vi "addNode.vi"(0 "reference":refnum<class "ImplicitParameterNode.lvclass">, 1 "node":refnum<class "AbstractNode.lvclass">, 2 "point2D":T1 {"y" format="%.2f"; "x" format="%.2f"}, 5 "error in (no error)":errorcluster) -> (14 "reference out":refnum<class "ImplicitParameterNode.lvclass">, 15 "add":bool, 19 "error out":errorcluster)   [LabVIEW 2014, in "ImplicitParameterNode.lvclass"]
doc: "public boolean addNode(Node n, Point2D p)"
uses:
  <resource>/Framework/Providers/Open_GDS/UML/ImplicitParameterNode_class/ImplicitParameterNode.lvclass
  <resource>/Framework/Providers/Open_GDS/UML/AbstractNode_class/AbstractNode.lvclass
  <resource>/Framework/Providers/Open_GDS/UML/General/Point/Point Point2D.ctl
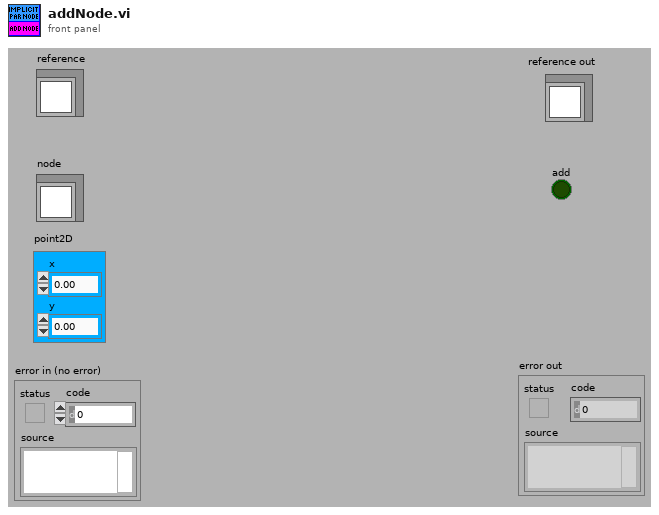
[diagram p1: front panel]
types:
  T1 = typedef "Point Point2D.ctl" = cluster{"x":dbl, "y":dbl}
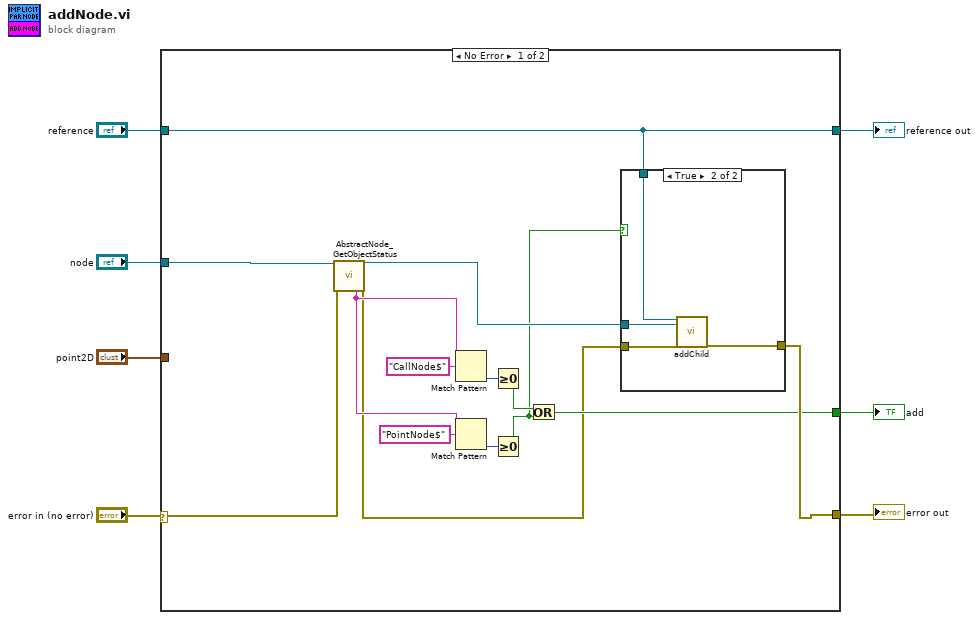
[diagram p0: block diagram]
diagram:
  n1 = case shown="No Error" "error in (no error)" {
    selector: "error in (no error)" -> [w19 w27]
    tunnel: "reference" -> [w21 w28]
    tunnel: [w20 w27] -> w6
    tunnel: [w21 w28] -> w5
    tunnel: "node" -> [w18 _]
    tunnel: "point2D" -> [_ _]
    tunnel: [w17 _] -> w1
    frame No Error {
      n2 = call <resource>:"AbstractNode_GetObjectStatus.vi"("reference in"=w18, "error in (no error)"=w19) -> ("Class name"=w14:string, "reference out"=w9:refnum<class "AbstractNode.lvclass">, "error out"=w10:errorcluster)  [unwired: 15 out]
      n3 = Match Pattern(string=w14, regular expression="CallNode$") -> (offset past match=w13:i32)  [unwired: 4 out]
      n4 = Match Pattern(string=w14, regular expression="PointNode$") -> (offset past match=w12:i32)  [unwired: 4 out]
      n5 = Greater Or Equal To 0?(x=w13) -> (x >= 0?=w11:bool)
      n6 = Greater Or Equal To 0?(x=w12) -> (x >= 0?=w8:bool)
      n7 = Or(x=w11, y=w8) -> (x .or. y?=w17:bool)
      n8 = case shown="True" w8 {
        tunnel: w10 -> [w22 w26]
        tunnel: [w22 w25] -> w20
        tunnel: w21 -> [_ w24]
        tunnel: w9 -> [_ w23]
        frame False {
        }
        frame True {
          n9 = call-dynamic "addChild.vi"("reference"=w24, "node"=w23, "error in (no error)"=w26) -> ("error out"=w25:errorcluster)  [unwired: 15 in, 1 out]
        }
      }
    }
    frame Error {
    }
  }
  "reference out" <- w5
  "error out" <- w6
  "add" <- w1
